vi "Deadband_Filter.vi"(9 "Deadband_Center":dbl=-0.00784 format="%#_13g", 10 "Input":dbl, 11 "Deadband_Size(%)":dbl=9.0 format="%#_13g") -> (3 "Deadbanded_Output":dbl)   [LabVIEW 2015]
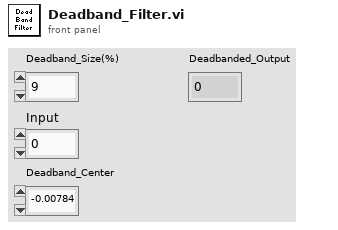
[diagram p1: front panel]
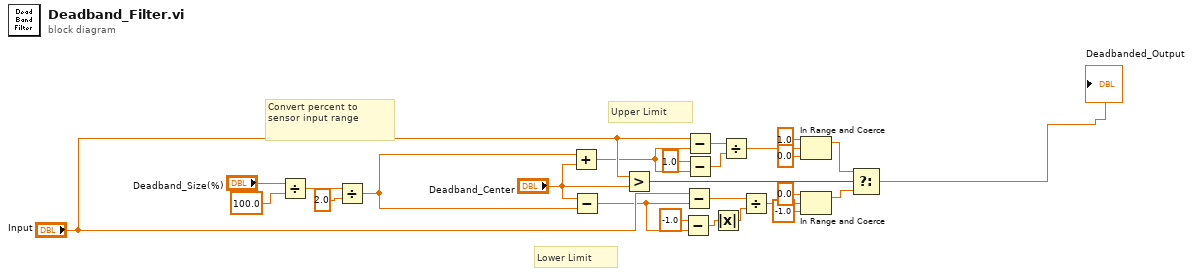
[diagram p0: block diagram]
diagram:
  # "Upper Limit"
  # "Lower Limit"
  # "Convert percent to\nsensor input range"
  n1 = Divide(x="Deadband_Size(%)", y=100.0) -> (x/y=w4:dbl)
  n2 = Divide(x=w4, y=2.0) -> (x/y=w5:dbl)
  n3 = Add(x=w5, y="Deadband_Center") -> (x+y=w8:dbl)
  n4 = Subtract(x="Deadband_Center", y=w5) -> (x-y=w17:dbl)
  n5 = Greater?(x="Input", y="Deadband_Center") -> (0:w24:bool)
  n6 = Subtract(x=-1.0, y=w17) -> (x-y=w25:dbl)
  n7 = Subtract(x="Input", y=w17) -> (x-y=w15:dbl)
  n8 = Subtract(x="Input", y=w8) -> (x-y=w9:dbl)
  n9 = Subtract(x=1.0, y=w8) -> (x-y=w10:dbl)
  n10 = Absolute Value(x=w25) -> (abs(x)=w26:dbl)
  n11 = Divide(x=w9, y=w10) -> (x/y=w13:dbl)
  n12 = Divide(x=w15, y=w26) -> (x/y=w18:dbl)
  n13 = In Range and Coerce(upper limit=1.0, x=w13, lower limit=0.0) -> (coerced(x)=w14:dbl)  [unwired: 1 out]
  n14 = In Range and Coerce(upper limit=0.0, x=w18, lower limit=-1.0) -> (coerced(x)=w21:dbl)  [unwired: 1 out]
  n15 = Select(t=w14, s=w24, f=w21) -> (s? t:f=→"Deadbanded_Output":dbl)
